vi "config.read.vi"(8 "error in":errorcluster) -> (0 "error out":errorcluster, 3 "paths":T1)   [LabVIEW 2024, in "Shared.lvlib"]
uses:
  Shared.lvlib
  <vilib>/addons/_JKI.lib/Serialization/JSON/JKI JSON Serialization.lvlib
  paths--cluster.ctl
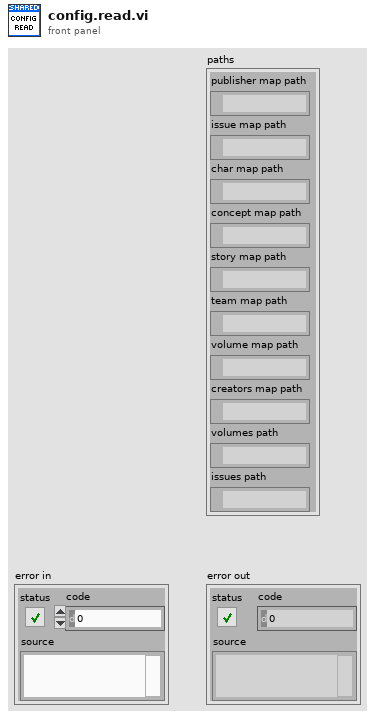
[diagram p1: front panel]
types:
  T1 = typedef "Shared.lvlib/paths--cluster.ctl" = cluster{"publisher map path":path, "issue map path":path, "char map path":path, "concept map path":path, "story map path":path, "team map path":path, "volume map path":path, "creators map path":path, "volumes path":path, "issues path":path}
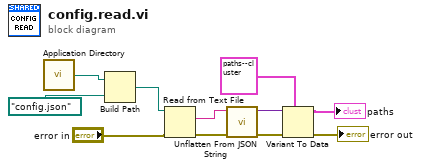
[diagram p0: block diagram]
diagram:
  n1 = call <vilib>:"Application Directory.vi"() -> ("Application Directory"=w11:path)
  n2 = Build Path(base path=w11, name or relative path=path "config.json") -> (appended path=w9:path)
  n3 = Read from Text File(file (use dialog)=w9, error in="error in") -> (text=w7:string, error out=w6:errorcluster)  [unwired: 2 in, 2 out]
  n4 = call <vilib>:"Unflatten From JSON String.vi"("error in"=w6, "JSON String"=w7) -> ("error out"=w3:errorcluster, "Variant"=w5:variant)  [unwired: 8 in]
  n5 = Variant To Data(error in=w3, type=T1 {"publisher map path"=path "", "issue map path"=path "", "char map path"=path "", "concept map path"=path "", "story map path"=path "", "team map path"=path "", "volume map path"=path "", "creators map path"=path "", "volumes path"=path "", "issues path"=path ""} ("paths"), Variant=w5) -> (data=→"paths":T1, error out=→"error out":errorcluster)
